vi "sv_VerifyAttributeName.vi"(5 "Attribute Name":string, 9 "error in (no error)":errorcluster, 13 "Data Type":string) -> (6 "Attribute Name Out":string, 10 "error out":errorcluster)   [LabVIEW 2017]
uses:
  <vilib>/Utility/error.llb/Error Cluster From Error Code.vi
  <vilib>/ErrorRing/Error Ring.xnode
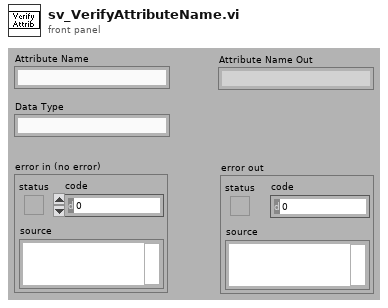
[diagram p1: front panel]
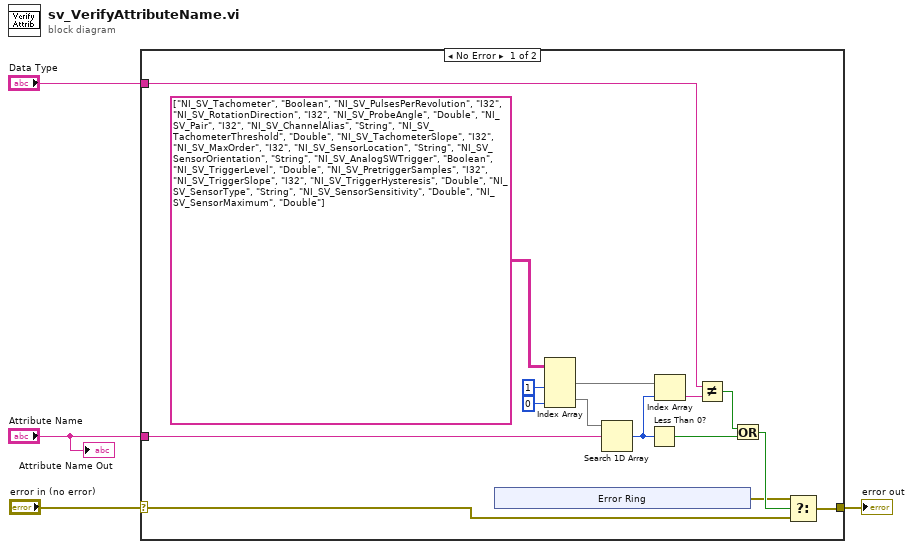
[diagram p0: block diagram]
diagram:
  n1 = case shown="No Error" "error in (no error)" {
    selector: "error in (no error)" -> [w19 w24]
    tunnel: [w18 w24] -> w3
    tunnel: "Attribute Name" -> [w17 _]
    tunnel: "Data Type" -> [w5 _]
    frame No Error {
      n2 = xnode "Error Ring"() -> ("error out"=w6:errorcluster)
      n3 = Index Array(array=string[][] [["NI_SV_Tachometer", "Boolean"], ["NI_SV_PulsesPerRevolution", "I32"], ["NI_SV_RotationDirection", "I32"], ["NI_SV_ProbeAngle", "Double"], ["NI_SV_Pair", "I32"], ["NI_SV_ChannelAlias", "String"], ["NI_SV_TachometerThreshold", "Double"], ["NI_SV_TachometerSlope", "I32"], ["NI_SV_MaxOrder", "I32"], ["NI_SV_SensorLocation", "String"], ["NI_SV_SensorOrientation", "String"], ["NI_SV_AnalogSWTrigger", "Boolean"], ["NI_SV_TriggerLevel", "Double"], ["NI_SV_PretriggerSamples", "I32"], ["NI_SV_TriggerSlope", "I32"], ["NI_SV_TriggerHysteresis", "Double"], ["NI_SV_SensorType", "String"], ["NI_SV_SensorSensitivity", "Double"], ["NI_SV_SensorMaximum", "Double"]], index (col) #1=1 ("index (row)"), index (col) #2=0 ("index (row)")) -> (element #1=w13:string[], element #2=w15:string[])  [unwired: 2 in]
      n4 = Search 1D Array(1D array=w15, element=w17) -> (index of element=w12:i32)  [unwired: 1 in]
      n5 = Less Than 0?(x=w12) -> (x < 0?=w11:bool)
      n6 = Index Array(array=w13, index=w12) -> (element=w10:string)
      n7 = Not Equal?(x=w5, y=w10) -> (x != y?=w9:bool)
      n8 = Or(x=w9, y=w11) -> (x .or. y?=w14:bool)
      n9 = Select(t=w6, s=w14, f=w19) -> (s? t:f=w18:errorcluster)
    }
    frame Error {
    }
  }
  "error out" <- w3
  "Attribute Name Out" <- "Attribute Name"
